vi "LS372_calculate_still_output.vi"(1 "Power (mW)":dbl, 2 "Resistance (Ohms)":dbl) -> (0 "Analog Output (%)":dbl)   [LabVIEW 2019]
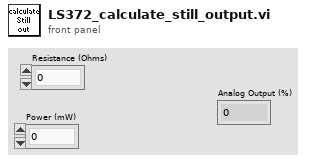
[diagram p1: front panel]
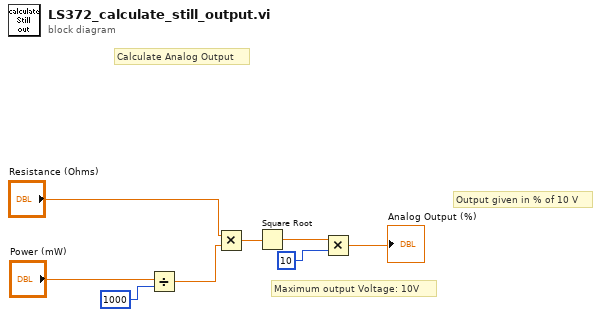
[diagram p0: block diagram]
diagram:
  # "Maximum output Voltage: 10V"
  # "Output given in % of 10 V"
  # "Calculate Analog Output"
  n1 = Divide(x="Power (mW)", y=1000) -> (x/y=w7:dbl)
  n2 = Multiply(x="Resistance (Ohms)", y=w7) -> (x*y=w4:dbl)
  n3 = Square Root(x=w4) -> (sqrt(x)=w3:dbl)
  n4 = Multiply(x=w3, y=10) -> (x*y=→"Analog Output (%)":dbl)
